vi "Open Debug File.vi"(4 "error in (no error)":errorcluster, 6 "App Name (\"\")":string, 7 "App Folder (Empty)":path) -> (0 "error out":errorcluster, 3 "Debug Ref":T1)   [LabVIEW 2011]
uses:
  <vilib>/Utility/config.llb/Config Data RefNum.ctl
  <vilib>/Utility/config.llb/NI_LVConfig.lvlib
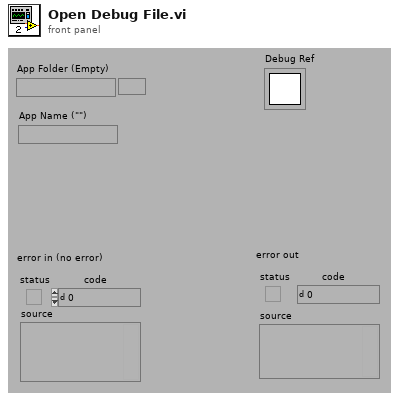
[diagram p1: front panel]
types:
  T1 = typedef "NI_LVConfig.lvlib/Config Data RefNum.ctl" = refnum<k1>
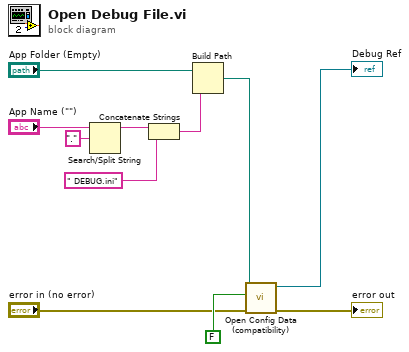
[diagram p0: block diagram]
diagram:
  n1 = Search/Split String(string="App Name (\"\")", search string/char (-)=".") -> (substring before match=w7:string)  [unwired: 3 out]
  n2 = Concatenate Strings(w7, " DEBUG.ini" ("search string/char (-)")) -> (w4:string)
  n3 = Build Path(base path="App Folder (Empty)", name or relative path=w4) -> (appended path=w3:path)
  n4 = call <vilib>:"Open Config Data (compatibility).vi"("error in (no error)"="error in (no error)", "create file if necessary (T)"=FALSE, "configuration file path"=w3) -> ("error out"=→"error out":errorcluster, "refnum"=→"Debug Ref":T1)  [unwired: 6 in, 1 out]
